vi "Prompted Inputs Configuration.vi"(6 "Write? (f)":bool, 7 "Connection Refnum":T2, 8 "error in (no error)":errorcluster, 9 "Configuration (\"\")":string, 11 "Template Keys (empty)":T1) -> (0 "error out":errorcluster, 1 "Configuration":string, 3 "Template Keys":T1, 5 "Connection Refnum":T2)   [LabVIEW 2011]
uses:
  Summitek EXT/ODBC/SQL Controls/Connection Refnum.ctl
  ITK EXT/utils/keyedarr.llb/Keyed Array.ctl
  ITK EXT/utils/strutil.llb/Case Matching.ctl
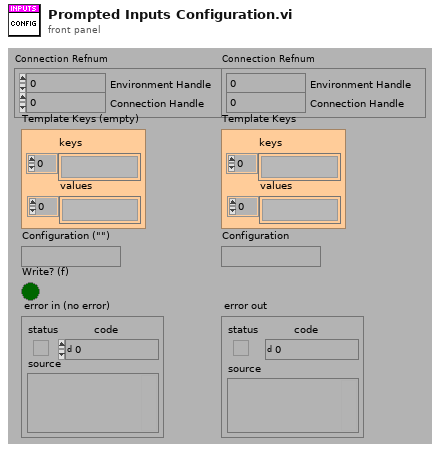
[diagram p1: front panel]
types:
  T1 = typedef "Keyed Array.ctl" = cluster{"keys":string[], "values":string[]}
  T2 = typedef "Connection Refnum.ctl" = cluster{"Environment Handle":i32, "Connection Handle":i32}
  T3 = typedef "Case Matching.ctl" = enum16{"a != A", "a == A", "system"}
  T4 = typedef "PI Test Parameters.ctl" = cluster{"Measurement":T5, "Limit":T6}
  T5 = typedef "PI Measurement Cluster.ctl" = cluster{"sxFieldId":string, "sValue":string, "nDataType":enum16{"Scalar", "Enumeration"}, "sUnits":string, "sDisplayName":string}
  T6 = typedef "PI Limit Parameters.ctl" = cluster{"Limits On":bool, "Limits":T7[]}
  T7 = typedef "PI Limit Definition.ctl" = cluster{"nComparison":T8, "sValue":string}
  T8 = typedef "PI Limit Comparison.ctl" = enum16{">", ">=", "<", "<=", "<>", "="}
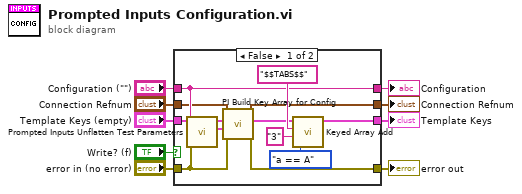
[diagram p0: block diagram]
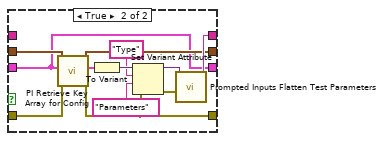
[diagram p2: hidden frame]
diagram:
  n1 = case shown="False" "Write? (f)" {
    tunnel: "error in (no error)" -> [w10 w27]
    tunnel: [w14 w22] -> w8
    tunnel: "Template Keys (empty)" -> [w12 w22]
    tunnel: "Configuration (\"\")" -> [w18 _]
    tunnel: [w13 w26] -> w5
    tunnel: [w18 w28] -> w4
    tunnel: "Connection Refnum" -> [w17 w25]
    tunnel: [w16 w24] -> w1
    frame False {
      n2 = call "Prompted Inputs Unflatten Test Parameters.vi"("error in (no error)"=w10, "Parameter String"=w18) -> ("Prompted Inputs Test Parameters"=w11:T4)  [unwired: 9 out]
      n3 = call "PI Build Key Array for Config.vi"("error in (no error)"=w10, "Prompted Inputs Test Parameters"=w11, "Template Keys (empty)"=w12, "Connection Refnum"=w17) -> ("error out"=w13:errorcluster, "new Template Keys"=w15:T1, "Connection Refnum"=w16:T2)  [unwired: 5 out]
      n4 = call "Keyed Array Add.vi"("case matching (sensitive)"=Case_Matching."a == A", "value"="3", "key"="$$TABS$$", "array in"=w15) -> ("array out"=w14:T1)  [unwired: 3 out]
    }
    frame True {
      n5 = call "PI Retrieve Key Array for Config.vi"("error in (no error)"=w27, "Key Array In"=w22, "Connection Refnum"=w25) -> ("error out"=w26:errorcluster, "Prompted Inputs Test Parameters"=w23:T4, "Connection Refnum"=w24:T2)  [unwired: 6 out]
      n6 = To Variant(anything=w23) -> (Variant=w33:variant)
      n7 = Set Variant Attribute(Variant=w33, name="Type", value="Parameters" ("name"), error in=w26) -> (Variant out=w29:variant, error out=w32:errorcluster)  [unwired: 1 out]
      n8 = call "Prompted Inputs Flatten Test Parameters.vi"("error in (no error)"=w32, "Parameter Variant"=w29) -> ("Parameter String"=w28:string)  [unwired: 9 out]
    }
  }
  "error out" <- w5
  "Connection Refnum" <- w1
  "Template Keys" <- w8
  "Configuration" <- w4
